vi "readHeader.vi"(8 "error in (no error)":errorcluster, 11 "M1M3SAL in":refnum<class "M1M3SAL.lvclass">) -> (0 "error out":errorcluster, 1 "Timeout":bool, 2 "Header":T1, 3 "M1M3SAL out":refnum<class "M1M3SAL.lvclass">)   [LabVIEW 2016, in "M1M3SupportCommunicator.lvlib" / "M1M3SAL.lvclass"]
uses:
  M1M3SAL.lvclass
  DataTypes/MessageHeader.ctl
  DataTypes/MessageTypes.ctl
  DataTypes/MessageTopics.ctl
  Common_RT_Utilities/U8ArrayParserAutoIndexing/U8ArrayParserAutoIndexing.lvclass
  M1M3SupportCommunicator.lvlib
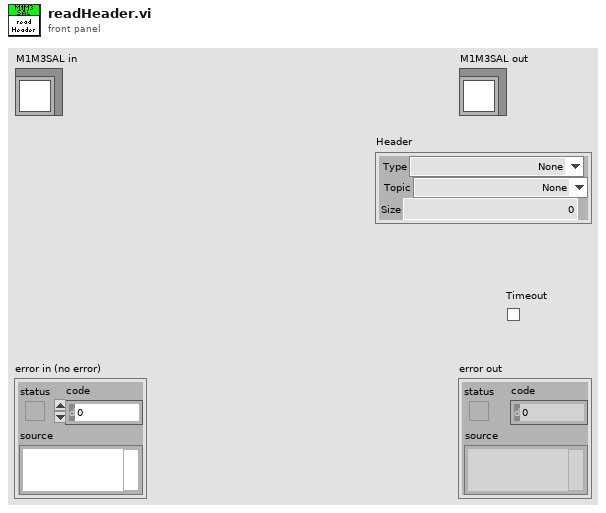
[diagram p1: front panel]
types:
  T1 = typedef "M1M3SupportCommunicator.lvlib/MessageHeader.ctl" = cluster{"Type":T2, "Topic":T3, "Size":i32}
  T2 = typedef "M1M3SupportCommunicator.lvlib/MessageTypes.ctl" = enum8{"None", "PutSample", "GetNextSample", "LogEvent", "GetEvent", "IssueCommand", "CommandId", "WaitForCompletion", "AcceptCommand", "AckCommand"}
  T3 = typedef "M1M3SupportCommunicator.lvlib/MessageTopics.ctl" = enum8{"None", "Start", "Enable", "Disable", "Standby", "AppliedSettingsMatchStart", "ErrorCode", "SettingVersions", "SummaryState", "DetailedState", "Exit"}
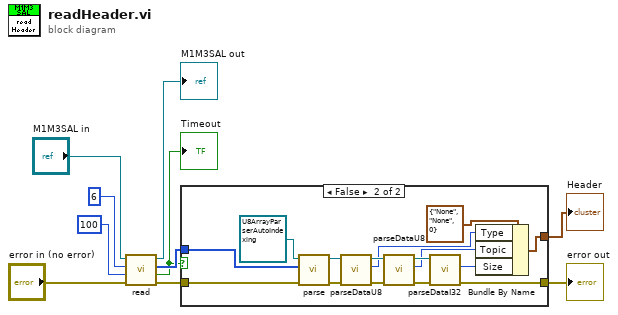
[diagram p0: block diagram]
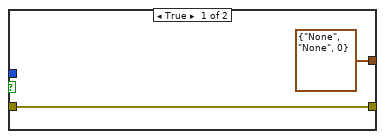
[diagram p2: hidden frame]
diagram:
  n1 = call "read.vi"("error in (no error)"="error in (no error)", "Timeout"=100, "NumberOfBytes"=6, "M1M3SAL in"="M1M3SAL in") -> ("error out"=w10:errorcluster, "Timeout"=w1:bool, "Data"=w9:u8[], "M1M3SAL out"=→"M1M3SAL out":refnum<class "M1M3SAL.lvclass">)  [unwired: 4 in]
  "Timeout" <- w1
  n2 = case shown="False" w1 {
    tunnel: w10 -> [w12 w24]
    tunnel: w9 -> [_ w19]
    tunnel: [T1 {"Type"=enum."None", "Topic"=enum."None", "Size"=0} ("Header") w14] -> w5
    tunnel: [w12 w13] -> w4
    frame True {
    }
    frame False {
      n3 = call "parse.vi"("error in (no error)"=w24, "Data"=w19, "U8ArrayParserAutoIndexing in"=refnum<class "U8ArrayParserAutoIndexing.lvclass"> refnum ("RTUtilities.lvlib:U8ArrayParserAutoIndexing.lvclass")) -> ("error out"=w25:errorcluster, "U8ArrayParserAutoIndexing out"=w21:refnum<class "U8ArrayParserAutoIndexing.lvclass">)  [unwired: 7 in]
      n4 = call "parseDataU8.vi"("error in (no error)"=w25, "U8ArrayParserAutoIndexing in"=w21) -> ("error out"=w26:errorcluster, "Data"=w17:u8, "U8ArrayParserAutoIndexing out"=w22:refnum<class "U8ArrayParserAutoIndexing.lvclass">)  [unwired: 7 in]
      n5 = call "parseDataU8.vi"("error in (no error)"=w26, "U8ArrayParserAutoIndexing in"=w22) -> ("error out"=w27:errorcluster, "Data"=w16:u8, "U8ArrayParserAutoIndexing out"=w23:refnum<class "U8ArrayParserAutoIndexing.lvclass">)  [unwired: 7 in]
      n6 = call "parseDataI32.vi"("error in (no error)"=w27, "U8ArrayParserAutoIndexing in"=w23) -> ("error out"=w13:errorcluster, "Data"=w15:i32)  [unwired: 7 in, 1 out]
      n7 = Bundle By Name(cluster=T1 {"Type"=enum."None", "Topic"=enum."None", "Size"=0} ("Header"), "Type"=w17, "Topic"=w16, "Size"=w15) -> (w14:T1)
    }
  }
  "error out" <- w4
  "Header" <- w5
